vi "Flush Buffer.vi"(8 "error in (no error)":errorcluster, 11 "Circular Buffer 2D U16 DVR Queue Circular Buffer in":refnum<class "Circular Buffer 2D U16 DVR Queue Circular Buffer.lvclass">) -> (0 "error out":errorcluster, 3 "Circular Buffer 2D U16 DVR Queue Circular Buffer out":refnum<class "Circular Buffer 2D U16 DVR Queue Circular Buffer.lvclass">)   [LabVIEW 2024, in "Circular Buffer 2D U16 DVR Queue Circular Buffer.lvclass"]
uses:
  Circular Buffer 2D U16 DVR Queue Circular Buffer.lvclass
  Circular Buffer 2D U16 DVR Queue Circular Buffer.lvclass/Circular Buffer 2D U16 DVR Queue Circular Buffer.ctl
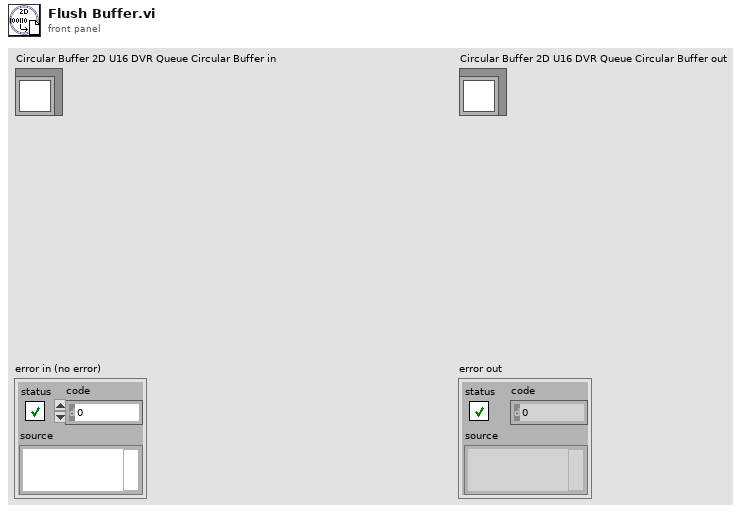
[diagram p1: front panel]
types:
  T1 = typedef "2D U16 DVR Queue.ctl" = refnum<queue>
  T2 = typedef "2D U16 DVR.ctl" = refnum<data-value>
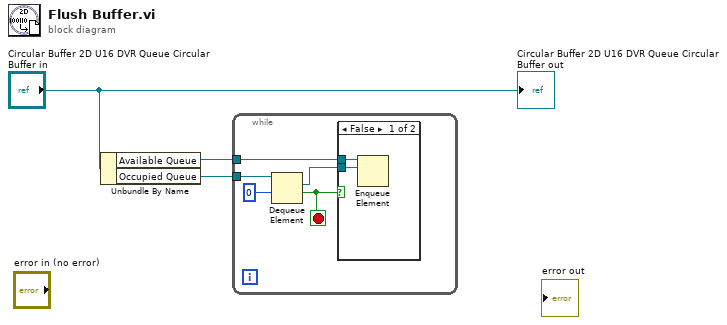
[diagram p0: block diagram]
diagram:
  n1 = Unbundle By Name("Circular Buffer 2D U16 DVR Queue Circular Buffer in") -> ("Available Queue"=w1:T1, "Occupied Queue"=w2:T1)
  n2 = while {
    tunnel: w2 -> [w8]
    tunnel: w1 -> [w6]
    stop <- w4 stop-if-true
    n3 = Dequeue Element(queue=w8, timeout in ms (-1)=0) -> (element=w5:T2, timed out?=w4:bool)  [unwired: 1 in, 2 out]
    n4 = case shown="False" w4 {
      tunnel: w6 -> [w10 _]
      tunnel: w5 -> [w9 _]
      frame False {
        n5 = Enqueue Element(queue=w10, element=w9) -> ()  [unwired: 2 in, 3 out]
      }
      frame True {
      }
    }
  }
  "Circular Buffer 2D U16 DVR Queue Circular Buffer out" <- "Circular Buffer 2D U16 DVR Queue Circular Buffer in"
